vi "DAQWaveformDataStore.vi"(3 "Error in":errorcluster, 4 "Experiment State":T1 {"RIO Settings"."Card Settings"."Sample Rate" format="%#_3p"; "Timing Settings"."Timing Channel Settings"."FrontPanelTime" format="%.3p"; "Timing Settings"."Timing Channel Settings"."Pulse width (s)" format="%.3p"; "Timing Settings"."Timing Channel Settings"."Delay (s)" format="%.3p"; "Digitizer Settings"."Card Settings"."Global Edge Type" items=["Rising"=10280, "Falling"=10171]; "Digitizer Settings"."Card Settings"."Sample Rate" format="%#_3p"}, 5 "Tree DVR In":refnum<data-value>) -> (0 "Error out":errorcluster)   [LabVIEW 2014]
uses:
  <vilib>/MDSplus/Classes/Tree_Class/Tree.lvclass
  Controls/ExperimentStateCluster.ctl
  Controls/DigitizerSettingsChannelSettings.ctl
  Controls/DigitizerSettingsCardSettingsArray.ctl
  Controls/DigitizerSettingsCardSettings.ctl
  Controls/TimingSettings.ctl
  Controls/TimingCardSettings.ctl
  Controls/TimingChannelSettings.ctl
  Controls/RIOSettingsExperimentStateCluster.ctl
  Controls/RIOSettingsChannelSettings.ctl
  Controls/RIOSettingsCardSettingsArray.ctl
  Controls/RIOSettingsCardSettings.ctl
  <vilib>/userdefined/High Color/nirio_resource_hc.ctl
  Controls/RIOData.ctl
  Controls/DIOChannel.ctl
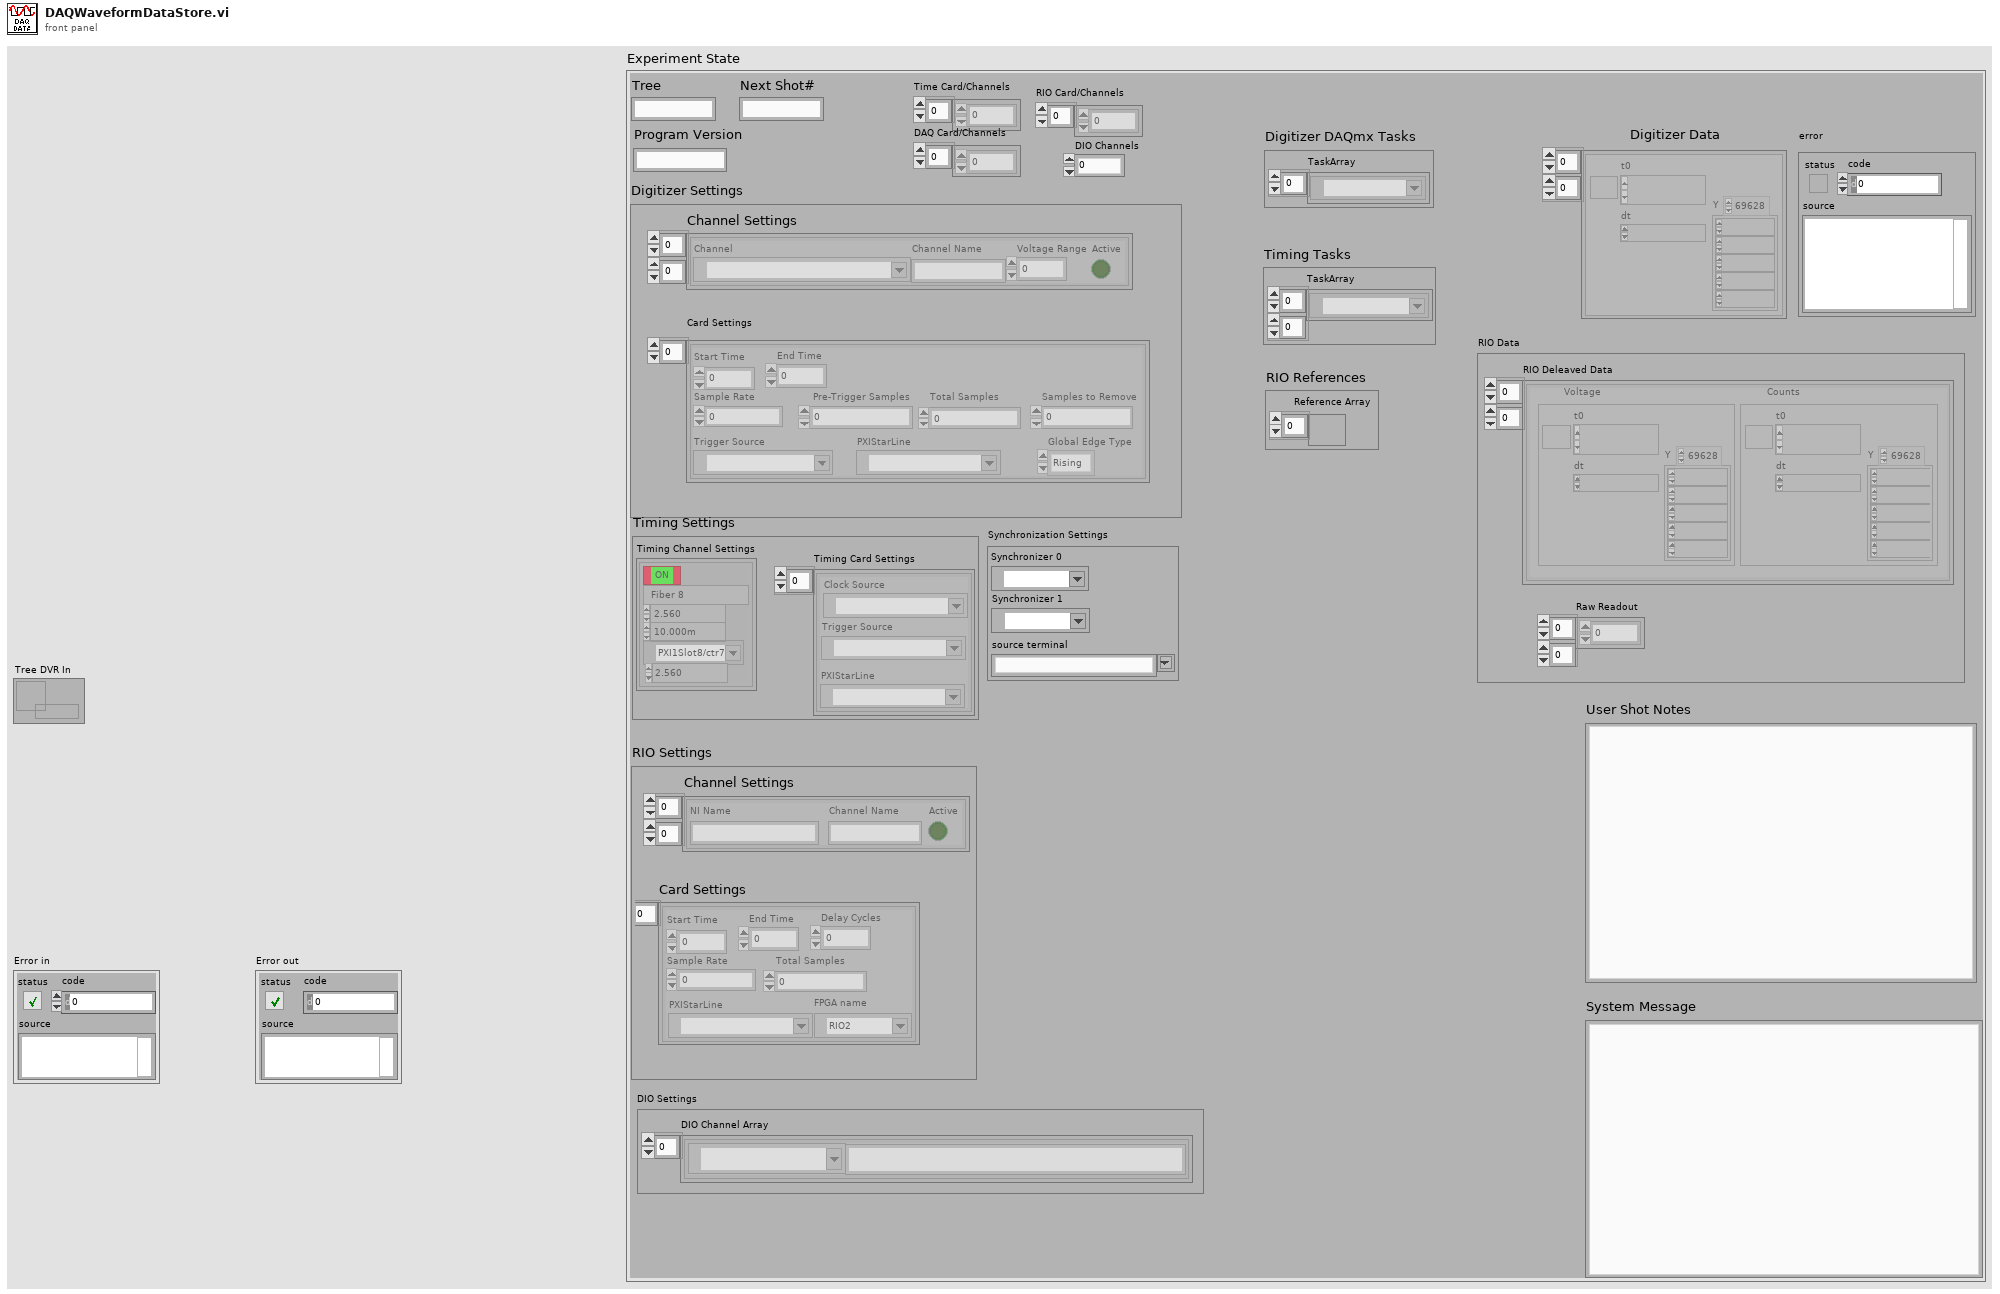
[diagram p1: front panel]
types:
  T1 = typedef "ExperimentStateCluster.ctl" = cluster{"error":errorcluster, "Digitizer DAQmx Tasks":cluster{"TaskArray":refnum<k21>[]}, "Digitizer Settings":cluster{"Channel Settings":T2[][], "Card Settings":T3}, "Synchronization Settings":cluster{"Synchronizer 0":refnum<k15>, "source terminal":string, "Synchronizer 1":refnum<k15>}, "Digitizer Data":waveform(dbl)[][], "Next Shot#":string, "System Message":string, "User Shot Notes":string, "Timing Settings":T5, "Timing Tasks":cluster{"TaskArray":refnum<k21>[][]}, "Tree":string, "Time Card/Channels":i32[], "DAQ Card/Channels":i32[], "Program Version":string, "RIO Settings":T8, "RIO References":cluster{"Reference Array":refnum<k20>[]}, "RIO Data":T13, "RIO Card/Channels":i32[], "DIO Channels":i32, "DIO Settings":cluster{"DIO Channel Array":T14[]}}
  T2 = typedef "DigitizerSettingsChannelSettings.ctl" = cluster{"Channel":tag, "Channel Name":string, "Voltage Range":dbl, "Active":bool}
  T3 = typedef "DigitizerSettingsCardSettingsArray.ctl" = T4[]
  T4 = typedef "DigitizerSettingsCardSettings.ctl" = cluster{"Start Time":dbl, "End Time":dbl, "Sample Rate":dbl, " Pre-Trigger Samples":u32, "Total Samples":i32, "Samples to Remove":u32, "Trigger Source":tag, "Global Edge Type":i32, "PXIStarLine":tag}
  T5 = typedef "TimingSettings.ctl" = cluster{"Timing Card Settings":T6[], "Timing Channel Settings":T7[][]}
  T6 = typedef "TimingCardSettings.ctl" = cluster{"Trigger Source":tag, "Clock Source":tag, "PXIStarLine":tag}
  T7 = typedef "TimingChannelSettings.ctl" = cluster{"Delay (s)":dbl, "Pulse width (s)":dbl, "Active":bool, "Channel Name":string, "counter":tag, "FrontPanelTime":dbl}
  T8 = typedef "RIOSettingsExperimentStateCluster.ctl" = cluster{"Channel Settings":T9[][], "Card Settings":T10}
  T9 = typedef "RIOSettingsChannelSettings.ctl" = cluster{"Channel Name":string, "Active":bool, "NI Name":string}
  T10 = typedef "RIOSettingsCardSettingsArray.ctl" = T11[]
  T11 = typedef "RIOSettingsCardSettings.ctl" = cluster{"Start Time":dbl, "End Time":dbl, "Sample Rate":dbl, "Total Samples":u64, "PXIStarLine":tag, "Delay Cycles":u64, "FPGA name":T12}
  T12 = typedef "nirio_resource_hc.ctl" = tag
  T13 = typedef "RIOData.ctl" = cluster{"RIO Deleaved Data":cluster{"Voltage":waveform(dbl), "Counts":waveform(i16)}[][], "Raw Readout":u64[][]}
  T14 = typedef "DIOChannel.ctl" = cluster{"Channel Name":string, "NI Name":tag}
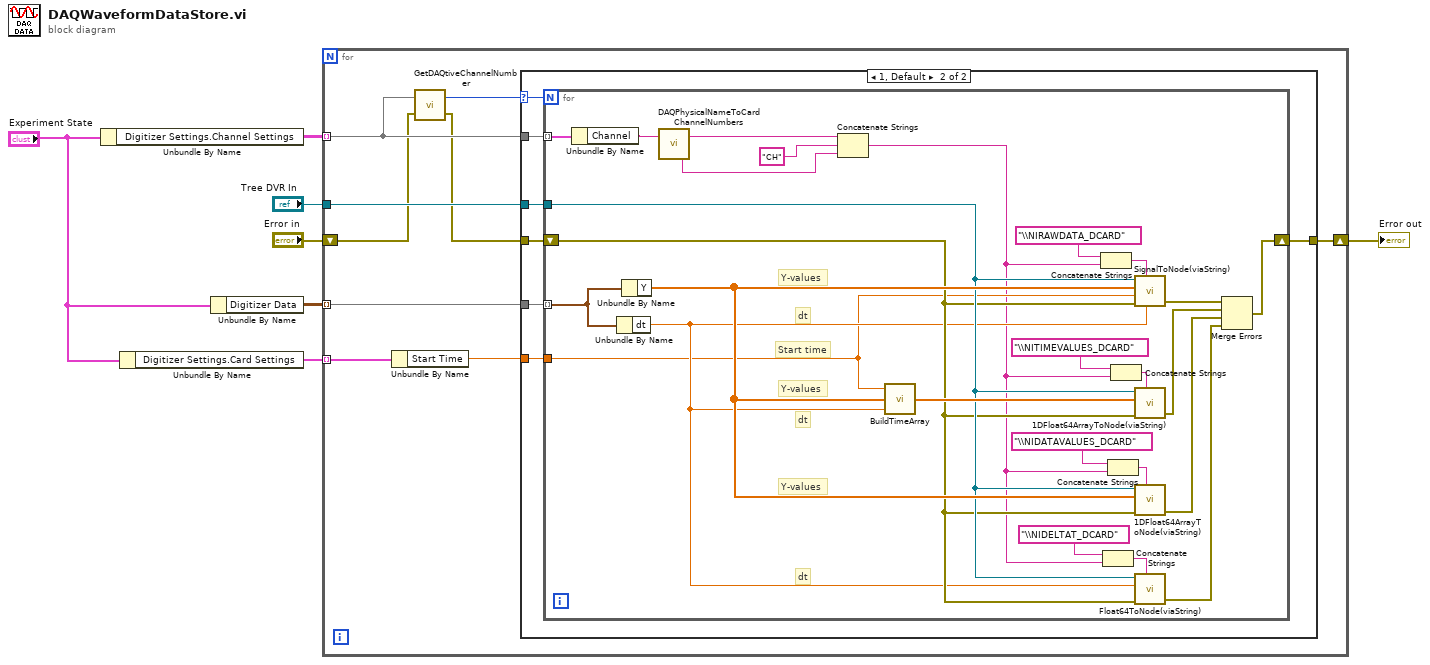
[diagram p0: block diagram]
diagram:
  n1 = Unbundle By Name("Experiment State") -> ("Digitizer Settings.Channel Settings"=w4:T2[][])
  n2 = Unbundle By Name("Experiment State") -> ("Digitizer Settings.Card Settings"=w3:T3)
  n3 = Unbundle By Name("Experiment State") -> ("Digitizer Data"=w1:waveform(dbl)[][])
  n4 = for {
    tunnel: "Tree DVR In" -> [w12]
    shift-right: [w13] -> w7
    shift-left: "Error in" -> [w10]
    tunnel: w1 -> [w14] mode=indexing
    tunnel: w3 -> [w16] mode=indexing
    tunnel: w4 -> [w11] mode=indexing
    n5 = Unbundle By Name(w16) -> ("Start Time"=w15:dbl)
    n6 = call "GetDAQtiveChannelNumber.vi"("error in (no error)"=w10, "Channel Settings"=w11) -> ("error out"=w9:errorcluster, "Numeric"=w8:i32)
    n7 = case shown="1, Default" w8 {
      selector: w8 -> [_ w18]
      tunnel: w15 -> [_ w24]
      tunnel: w14 -> [_ w23]
      tunnel: [w17 w22] -> w13
      tunnel: w12 -> [_ w21]
      tunnel: w11 -> [_ w20]
      tunnel: w9 -> [w17 w19]
      frame 0 {
      }
      frame 1, Default {
        n8 = for {
          N: w18 -> [_]
          tunnel: w23 -> [w50] mode=indexing
          tunnel: w21 -> [w38]
          shift-right: [w47] -> w22
          shift-left: w19 -> [w37]
          tunnel: w24 -> [w34]
          tunnel: w20 -> [w33] mode=indexing
          # "dt"
          # "dt"
          # "Y-values"
          # "Y-values"
          # "Y-values"
          # "dt"
          # "Start time"
          n9 = Unbundle By Name(w33) -> ("Channel"=w32:tag)
          n10 = Unbundle By Name(w50) -> ("dt"=w36:dbl)
          n11 = Unbundle By Name(w50) -> ("Y"=w41:dbl[])
          n12 = call "DAQPhysicalNameToCardChannelNumbers.vi"("NI Physical Channel"=w32) -> ("Channel #"=w30:string, "Card #"=w31:string)  [unwired: 1 in]
          n13 = Concatenate Strings(w31, "CH" ("string"), w30) -> (w25:string)
          n14 = call "BuildTimeArray.vi"("Time Increment (dt)"=w36, "Data Array (y-values)"=w41, "Start Time (t_o)"=w34) -> ("Time Array (x-values)"=w44:dbl[])
          n15 = Concatenate Strings("\\NIRAWDATA_DCARD" ("string"), w25) -> (w46:string)
          n16 = Concatenate Strings("\\NIDELTAT_DCARD" ("string"), w25) -> (w39:string)
          n17 = Concatenate Strings("\\NIDATAVALUES_DCARD" ("string"), w25) -> (w42:string)
          n18 = Concatenate Strings("\\NITIMEVALUES_DCARD" ("string"), w25) -> (w45:string)
          n19 = call "SignalToNode(viaString).vi"("Tree DVR in"=w38, "NodePath"=w46, "y-axis (Data Range)"=w41, "Start Time"=w34, "Delta t"=w36, "Error in"=w37) -> ("Error out"=w48:errorcluster)  [unwired: 1 in, 1 out]
          n20 = call "1DFloat64ArrayToNode(viaString).vi"("Tree DVR in"=w38, "DBL Array"=w44, "error in (no error)"=w37, "NodePath"=w45) -> ("error out"=w43:errorcluster)  [unwired: 2 in, 1 out]
          n21 = call "1DFloat64ArrayToNode(viaString).vi"("Tree DVR in"=w38, "DBL Array"=w41, "error in (no error)"=w37, "NodePath"=w42) -> ("error out"=w40:errorcluster)  [unwired: 2 in, 1 out]
          n22 = call "Float64ToNode(viaString).vi"("Tree DVR in"=w38, "DBL in"=w36, "error in"=w37, "NodePath"=w39) -> ("error out"=w35:errorcluster)  [unwired: 2 in, 1 out]
          n23 = Merge Errors(w48, w43, w40, w35) -> (w47:errorcluster)
        }
      }
    }
  }
  "Error out" <- w7
